vi "CompressToCBZ.vi"(7 "Clean Filename?":bool, 8 "error in":errorcluster, 9 "Abort?":bool, 10 "FormerFilename":path, 11 "Working Path":path) -> (0 "error out":errorcluster, 2 "NewFilename":path, 3 "Working Path Out":path)   [LabVIEW 2024]
uses:
  <userlib>/_OpenG.lib/file/file.llb/Convert File Extension (Path)__ogtk.vi
  <userlib>/_OpenG.lib/file/file.llb/openg_file.lvlib
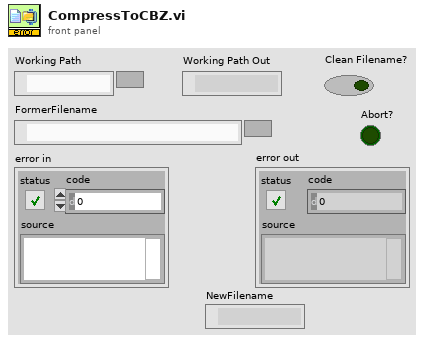
[diagram p1: front panel]
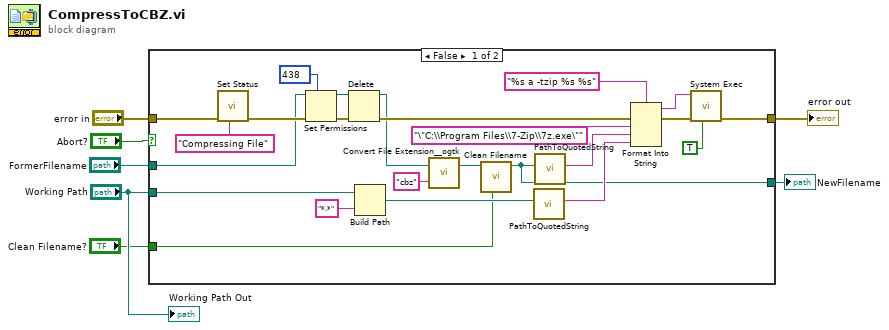
[diagram p0: block diagram]
diagram:
  n1 = case shown="False" "Abort?" {
    tunnel: [w25 w32] -> w7
    tunnel: "FormerFilename" -> [w10 _]
    tunnel: "error in" -> [w15 w32]
    tunnel: "Working Path" -> [w20 _]
    tunnel: "Clean Filename?" -> [w16 _]
    tunnel: [w8 _] -> w1
    frame False {
      n2 = call "Set Status.vi"("Status Message"="Compressing File" ("Value"), "error in (no error)"=w15) -> ("error out"=w12:errorcluster)  [unwired: 9 in]
      n3 = Set Permissions(7:i16 438 ("permissions"), 8:w12, 11:w10) -> (0:w11:errorcluster, 3:w9:path)  [unwired: 2 in]
      n4 = Delete(path (use dialog)=w9, error in=w11) -> (deleted path=w22:path, error out=w23:errorcluster)  [unwired: 3 in, 1 out]
      n5 = Build Path(base path=w20, name or relative path="*.*") -> (appended path=w18:path)
      n6 = call-poly <userlib>:"Convert File Extension__ogtk.vi"("new ending (none)"="cbz", "file name"=w22) -> ("new filename"=w17:path)  [unwired: 1 out]
      n7 = call "Clean Filename.vi"("Clean Filename?"=w16, "Filepath in"=w17) -> ("Filepath out"=w8:path)  [unwired: 8 in, 1 out]
      n8 = call "PathToQuotedString.vi"("Path"=w18) -> ("String"=w21:string)  [unwired: 10 in]
      n9 = call "PathToQuotedString.vi"("Path"=w8) -> ("String"=w28:string)  [unwired: 10 in]
      n10 = Format Into String(format string="%s a -tzip %s %s", error in=w23, "\"C:\\Program Files\\7-Zip\\7z.exe\"" ("input 1"), w28, w21) -> (resulting string=w27:string, error out=w26:errorcluster)  [unwired: 1 in]
      n11 = call <vilib>:"System Exec.vi"("run minimized? (F)"=TRUE, "error in (no error)"=w26, "command line"=w27) -> ("error out"=w25:errorcluster)  [unwired: 5 in, 3 out]
    }
    frame True {
    }
  }
  "error out" <- w7
  "NewFilename" <- w1
  "Working Path Out" <- "Working Path"
